vi "SelectPatternFilePath.vi"(8 "Error In":errorcluster, 11 "Start Path":path=path "" caption="start path") -> (0 "Error Out":errorcluster, 2 "Cancelled?":bool, 3 "Pattern Path":path)   [LabVIEW 2012, in "Virtual-PGA.lvlib"]
doc: "This VI displays a dialog for selecting a XML file to load as a pattern."
uses:
  Virtual-PGA.lvlib
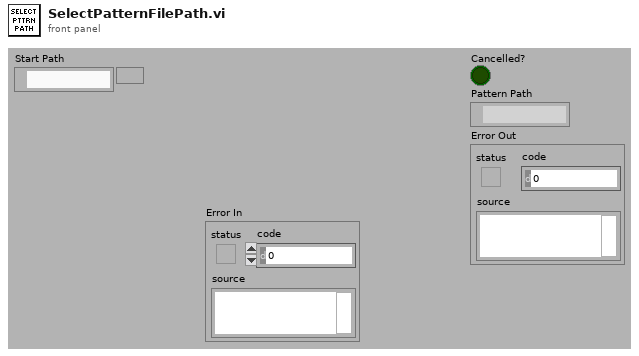
[diagram p1: front panel]
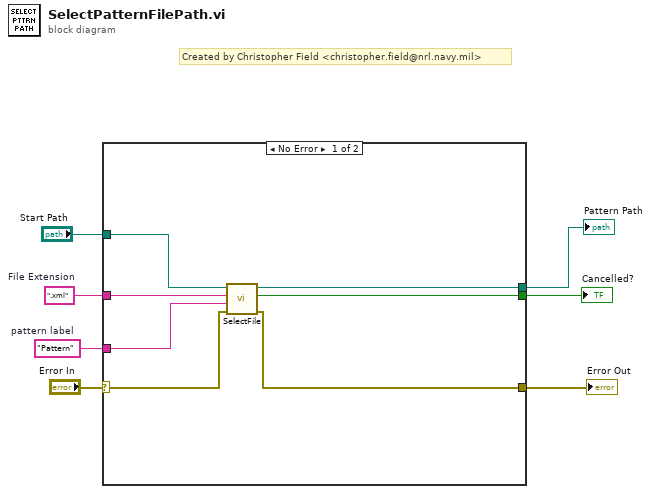
[diagram p0: block diagram]
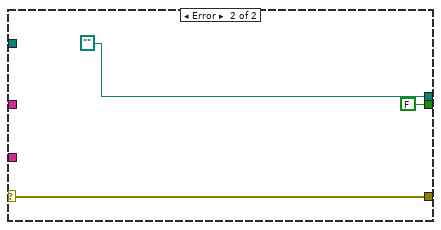
[diagram p2: hidden frame]
diagram:
  w6 = ".xml"  # File Extension
  w5 = "Pattern"  # pattern label
  # "Created by Christopher Field <christopher.field@nrl.navy.mil>"
  n1 = case shown="No Error" "Error In" {
    selector: "Error In" -> [w11 w17]
    tunnel: "Start Path" -> [w8 _]
    tunnel: w6 -> [w9 _]
    tunnel: w5 -> [w10 _]
    tunnel: [w14 path ""] -> w4
    tunnel: [w13 FALSE ("Cancelled?")] -> w3
    tunnel: [w12 w17] -> w2
    frame No Error {
      n2 = call "SelectFile.vi"("Error In"=w11, "File Description"=w10, "File Extension (.*)"=w9, "Start Path"=w8) -> ("Error Out"=w12:errorcluster, "Cancelled?"=w13:bool, "Selected File Path"=w14:path)  [unwired: 5 in]
    }
    frame Error {
    }
  }
  "Cancelled?" <- w3
  "Pattern Path" <- w4
  "Error Out" <- w2
